vi "ukol 2.vi"() -> ()   [LabVIEW 2023]
uses:
  <vilib>/addons/Digital Filter Design/Process.llb/DFD Filtering (Wfm).vi
  <vilib>/measure/NI_MABase.lvlib
  <vilib>/addons/Digital Filter Design/NI_DigFilterLicensed.lvlib
panel:
  out "Waveform Graph 6":waveform(dbl)[](graph)
  out "Waveform Graph 5":waveform(dbl)[](graph)
  out "Waveform Graph 4":waveform(dbl)[](graph)
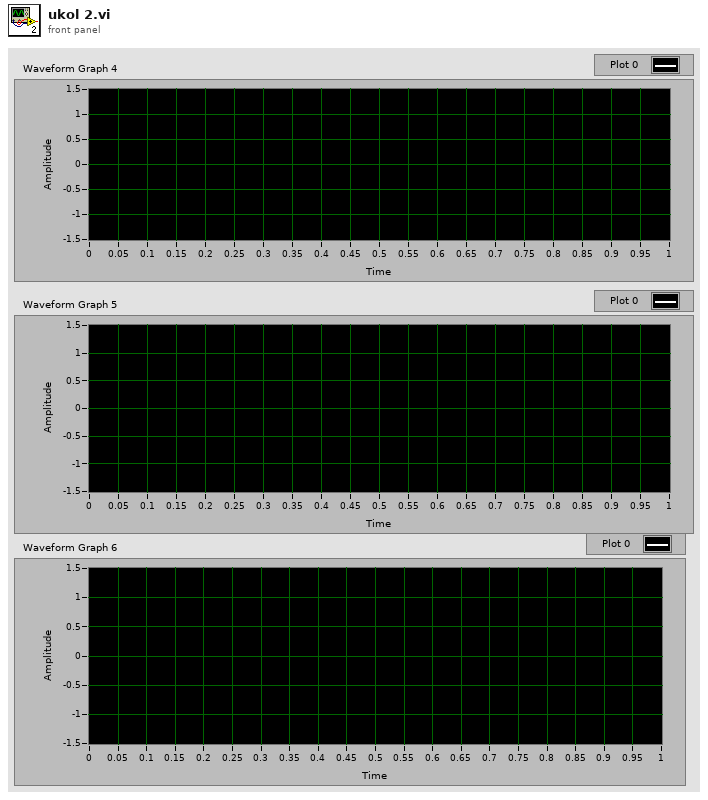
[diagram p1: front panel]
types:
  T1 = typedef "NI_DigFilterLicensed.lvlib/DFD Filter Obj.ctl" = cluster{"mSRate_Fs":dbl, "mSRate_Version":string, "mSRate_Comments":string, "mSRate_OrgCoef":T2, "mSRate_CurCoef":T2, "mSRate_Quantized?":bool, "mSRate_QCoef":T2, "mSRate_QSettings":T4[], "mSRate_Order":i32, "mSRate_Scaling":cluster{"mSRate_ScaleByPowerOf2?":bool, "mSRate_ScaleType":T6}}
  T2 = typedef "NI_DigFilterLicensed.lvlib/DFD Filter Coef.ctl" = cluster{"type":T3, "gain":dbl, "coef a (k)":dbl[], "coef b (v)":dbl[]}
  T3 = typedef "NI_DigFilterLicensed.lvlib/DFD Filter Structure Type Selector.ctl" = enum16{"Undefined", "FIR Direct Form", "FIR Direct Form Transposed", "FIR Symmetric", "FIR Antisymmetric", "IIR Direct Form I", "IIR Direct Form I Transposed", "IIR Direct Form II", "IIR Direct Form II Transposed", "IIR Cascaded Second Order Sections Form I", "IIR Cascaded Second Order Sections Form I Transposed", "IIR Cascaded Second Order Sections Form II", "IIR Cascaded Second Order Sections Form II Transposed", "Lattice Allpass (basic sections)", "Lattice Allpass (one multiplier sections)", "Lattice Allpass (normalized sections)", "Lattice AR (basic sections)", "Lattice AR (one multiplier sections)", "Lattice AR (normalized sections)", "Lattice MA (minimum phase)", "Lattice MA (maximum phase)", "Lattice ARMA (basic sections)", "Lattice ARMA (one multiplier sections)", "Lattice ARMA (normalized sections)"}
  T4 = typedef "NI_DigFilterLicensed.lvlib/dfd_Internal Quantization Settings.ctl" = cluster{"source":T5, "wl":i16, "iwl":i16, "overflow mode":enum16{"Saturation", "Wrap"}, "rounding mode":enum16{"Nearest", "Truncation"}, "signed?":bool}
  T5 = typedef "NI_DigFilterLicensed.lvlib/dfd_Internal Quantization Srcs.ctl" = u16
  T6 = typedef "NI_DigFilterLicensed.lvlib/DFD Coef Norm Type.ctl" = enum16{"No Norm", "Time Domain 1-Norm", "Time Domain 2-Norm", "Time Domain Inf-Norm"}
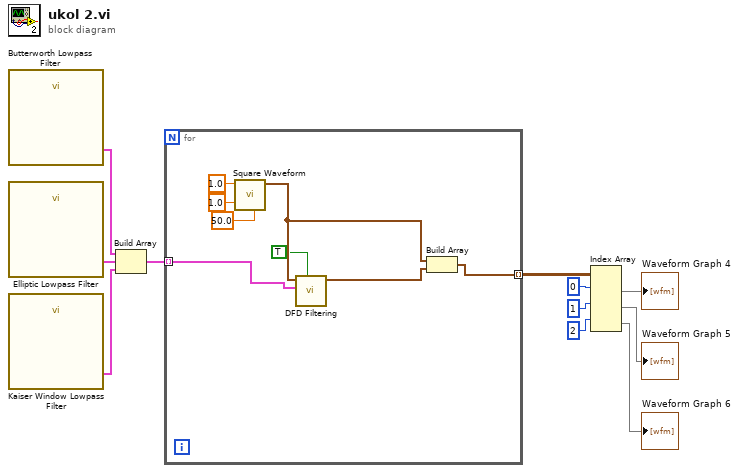
[diagram p0: block diagram]
diagram:
  n1 = call "Butterworth Lowpass Filter"() -> ("filter out"=w11:T1)  [unwired: 10 in, 1 out]
  n2 = call "Elliptic Lowpass Filter"() -> ("filter out"=w10:T1)  [unwired: 10 in, 1 out]
  n3 = call "Kaiser Window Lowpass Filter"() -> ("filter out"=w9:T1)  [unwired: 10 in, 1 out]
  n4 = Build Array(w11, w10, w9) -> (w8:T1[])
  n5 = for {
    tunnel: w8 -> [w16] mode=indexing
    tunnel: [w13] -> w1 mode=indexing
    n6 = call <vilib>:"Square Waveform.vi"("duty cycle (%)"=50.0, "amplitude"=1.0, "frequency"=1.0) -> ("signal out"=w15:waveform(dbl))  [unwired: 7 in, 1 out]
    n7 = call-poly <vilib>:"DFD Filtering.vi"("init? (F)"=TRUE, "filter"=w16, "signal in"=w15) -> ("signal out"=w14:waveform(dbl))  [unwired: 7 in, 1 out]
    n8 = Build Array(w15, w14) -> (w13:waveform(dbl)[])
  }
  n9 = Index Array(array=w1, index (row) #1=0 ("index"), index (row) #2=1 ("index"), index (row) #3=2 ("index")) -> (element #1=→"Waveform Graph 4":waveform(dbl)[], element #2=→"Waveform Graph 5":waveform(dbl)[], element #3=→"Waveform Graph 6":waveform(dbl)[])  [unwired: 3 in]
